vi "DriveGetSwerveKinematics.vi"() -> (0 "SWERVE_DRIVE_KINEMATICS":T1 {"SavedModuleStates"."Angle"."SIN" format="%13.4f"; "SavedModuleStates"."Angle"."COS" format="%13.4f"; "SavedModuleStates"."Angle"."VALUE" format="%13.4f"; "PrevCoR"."Y" format="%14.3f"; "PrevCoR"."X" format="%14.3f"; "Modules"."Y" format="%14.3f"; "Modules"."X" format="%14.3f"})   [LabVIEW 2020]
uses:
  <vilib>/Rock Robotics/WPI/ThirdParty/JAS_Junk/TrajLib/TypeDef/SWERVE_DRIVE_KINEMATICS.ctl
  <vilib>/Analysis/Matrix/Datatypes/RealMatrix.ctl
  <vilib>/Rock Robotics/WPI/ThirdParty/JAS_Junk/TrajLib/TypeDef/TRANSLATION2D.ctl
  <vilib>/Rock Robotics/WPI/ThirdParty/JAS_Junk/TrajLib/TypeDef/SWERVE_DRIVE_MODULE_STATE.ctl
  <vilib>/Rock Robotics/WPI/ThirdParty/JAS_Junk/TrajLib/TypeDef/ROTATION2D.ctl
  DriveGlobal.vi
  <vilib>/Analysis/Matrix/NI_Matrix.lvlib
  <vilib>/Rock Robotics/WPI/ThirdParty/JAS_Junk/TrajLib/Trajectory_Library.lvlib
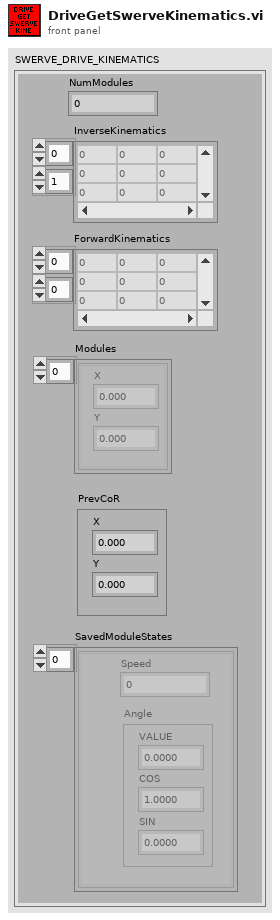
[diagram p1: front panel]
types:
  T1 = typedef "Trajectory_Library.lvlib/SWERVE_DRIVE_KINEMATICS.ctl" = cluster{"NumModules":i32, "InverseKinematics":T2, "ForwardKinematics":T2, "Modules":T3[], "PrevCoR":T3, "SavedModuleStates":T4[]}
  T2 = typedef "NI_Matrix.lvlib/RealMatrix.ctl" = dbl[][]
  T3 = typedef "Trajectory_Library.lvlib/TRANSLATION2D.ctl" = cluster{"X":dbl, "Y":dbl}
  T4 = typedef "Trajectory_Library.lvlib/SWERVE_DRIVE_MODULE_STATE.ctl" = cluster{"Speed":dbl, "Angle":T5}
  T5 = typedef "Trajectory_Library.lvlib/ROTATION2D.ctl" = cluster{"VALUE":dbl, "COS":dbl, "SIN":dbl}
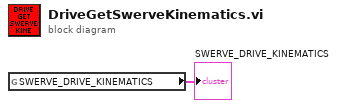
[diagram p0: block diagram]
diagram:
  n1 = global read "DriveGlobal.vi" "SWERVE_DRIVE_KINEMATICS"() -> (→"SWERVE_DRIVE_KINEMATICS":T1)
